vi "DisplayCurrentValues.vi"(8 "error in (no error)":errorcluster) -> (0 "error out":errorcluster, 1 "PDP Energy (J)":dbl, 2 "PDP Current (A)":dbl[](array[numeric]), 3 "Sum of Current":dbl, 4 "PDP Power (W)":dbl)   [LabVIEW 2019]
uses:
  <vilib>/Rock Robotics/Network Tables/NT Write Numeric Array.vi
panel:
  out "PDP Wattage":dbl[](array[numeric])
  out "voltage (V)":dbl
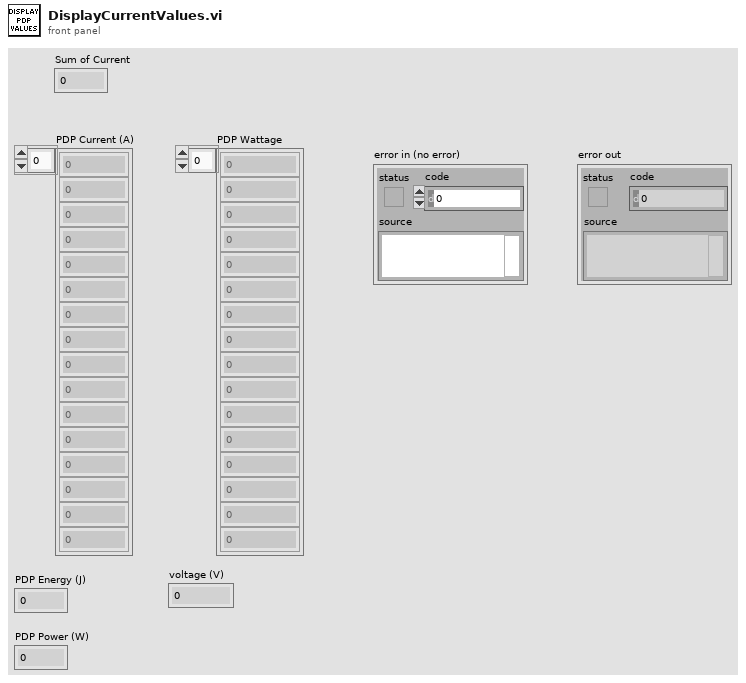
[diagram p1: front panel]
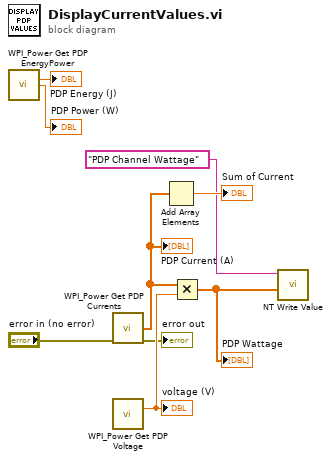
[diagram p0: block diagram]
diagram:
  n1 = call <vilib>:"WPI_Power Get PDP EnergyPower.vi"() -> ("Energy (J)"=→"PDP Energy (J)":dbl, "Power (W)"=→"PDP Power (W)":dbl)  [unwired: 13 in, 1 out]
  n2 = call <vilib>:"WPI_Power Get PDP Currents.vi"("error in"="error in (no error)") -> ("all currents (A)"=w6:dbl[], "error out"=→"error out":errorcluster)  [unwired: 12 in, 1 out]
  "PDP Current (A)" <- w6
  n3 = call <vilib>:"WPI_Power Get PDP Voltage.vi"() -> ("voltage (V)"=w5:dbl)  [unwired: 14 in, 1 out]
  "voltage (V)" <- w5
  n4 = Add Array Elements(numeric array=w6) -> (sum=→"Sum of Current":dbl)
  n5 = Multiply(x=w6, y=w5) -> (x*y=w4:dbl[])
  "PDP Wattage" <- w4
  n6 = call-poly <vilib>:"NT Write Value.vi"("Numeric Array"=w4, "Name"="PDP Channel Wattage") -> ()  [unwired: 9 in, 1 out]
